vi "Get Supported Targets.vi"(8 "error in":errorcluster, 11 "Tag Bus Web Interface configuration in":refnum<class "Tag Bus Web Interface configuration.lvclass">) -> (0 "error out":errorcluster, 2 "supported targets":T1[](array[typedef]), 3 "Tag Bus Web Interface configuration out":refnum<class "Tag Bus Web Interface configuration.lvclass">)   [LabVIEW 2013, in "Tag Bus Web Interface configuration.lvclass"]
doc: "Provides an interface for determining the targets supported by a given module configuration/runtime class pairing. This should be overridden by any useful child class."
uses:
  Tag Bus Web Interface configuration.lvclass
  <vilib>/NI/Tag Bus Module Framework/root configuration/Target Types.ctl
  <vilib>/NI/Tag Bus Module Framework/root configuration/TBM configuration.lvclass
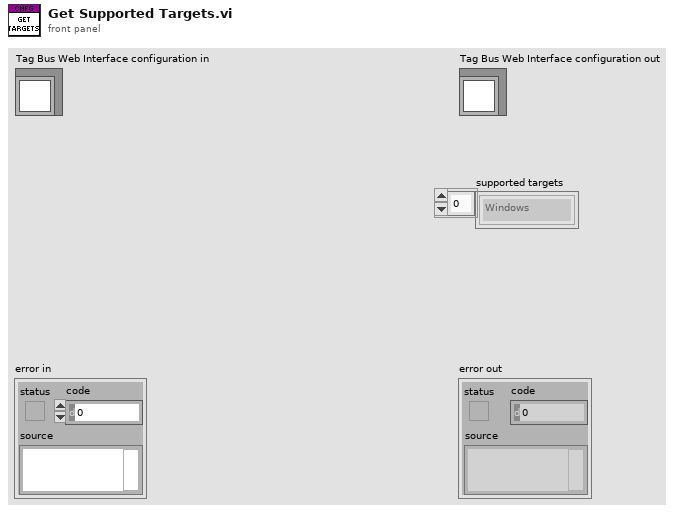
[diagram p1: front panel]
types:
  T1 = typedef "TBM configuration.lvclass/Target Types.ctl" = enum16{"Windows", "Mac", "Linux", "Linux RT", "VxWorks", "Pharlap", "Other"}
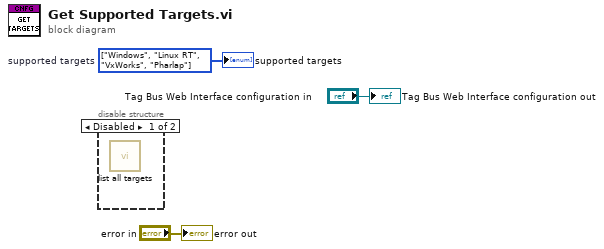
[diagram p0: block diagram]
diagram:
  w1 = T1[] [enum."Windows", enum."Linux RT", enum."VxWorks", enum."Pharlap"] items=["Windows", "Mac", "Linux", "Linux RT", "VxWorks", "Pharlap", "Other"]  # supported targets
  n1 = disable-structure shown="Disabled" {
    frame Disabled {
      n2 = call <vilib>:"list all targets.vi"() -> ()  [unwired: 11 in, 1 out]
    }
    frame Enabled {
    }
  }
  "error out" <- "error in"
  "Tag Bus Web Interface configuration out" <- "Tag Bus Web Interface configuration in"
  "supported targets" <- w1
